vi "Z_HSw.vi"(8 "error in (no error)":errorcluster, 10 "Z_Source":T1, 11 "Z_HSw_in":refnum<class "Z_HSw.lvclass">) -> (0 "error out":errorcluster, 3 "Z_HSw_out":refnum<class "Z_HSw.lvclass">)   [LabVIEW 2019, in "Z_HSw.lvclass"]
uses:
  Z_HSw.lvclass
  ctl/Z_SourceInd.ctl
  ctl/Z_SourceIndL.ctl
  Z_source.ctl
  Z_HSw.lvclass/Z_HSw.ctl
  ctl/Z_HSw_state.ctl
  Timer Delay/Timers.lvlib
panel:
  out "Z1 ind":T2
  out "Z1 ind 2":T3
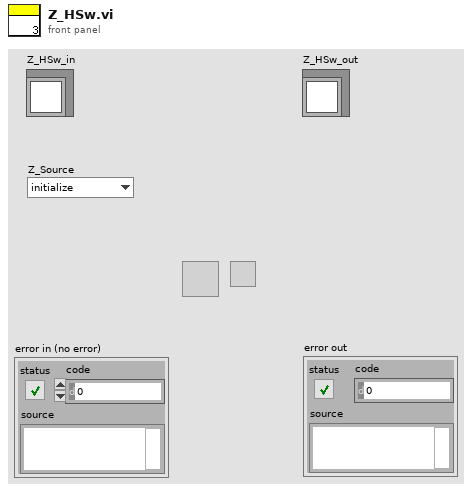
[diagram p1: front panel]
types:
  T1 = typedef "Z_source.ctl" = enum8{"initialize", "local disabled", "local hand", "hand", "auto", "dist"}
  T2 = typedef "Z_HSw.lvclass/Z_SourceIndL.ctl" = u8
  T3 = typedef "Z_HSw.lvclass/Z_SourceInd.ctl" = u8
  T4 = typedef "Z_HSw.lvclass/Z_HSw_state.ctl" = enum16{"init", "switch hand", "not hand", "hand", "switch auto", "not auto", "auto"}
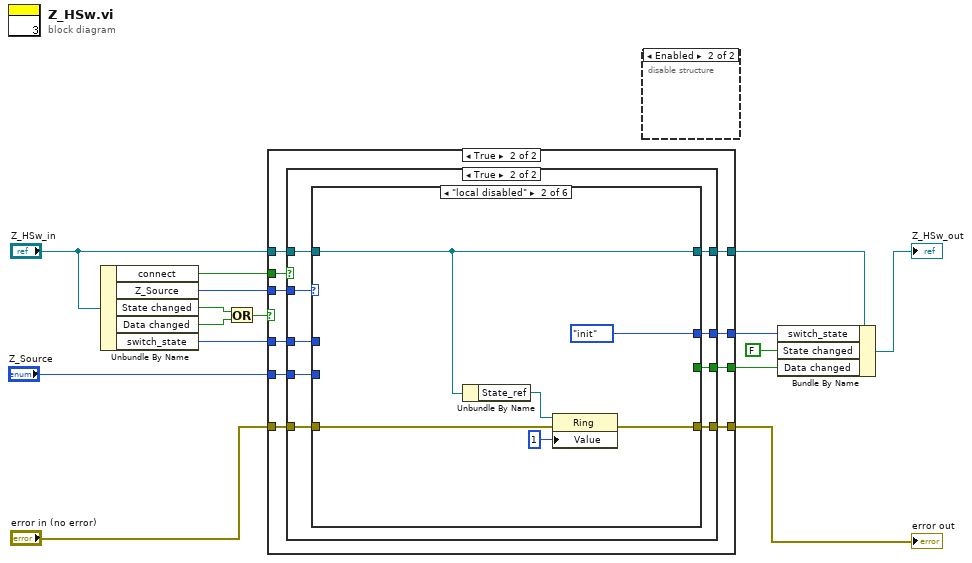
[diagram p0: block diagram]
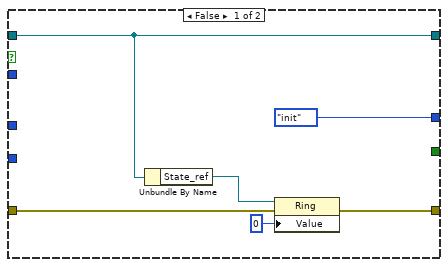
[diagram p3: hidden frame]
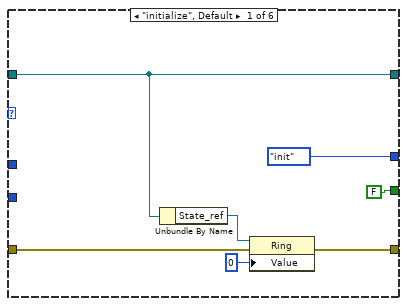
[diagram p4: hidden frame]
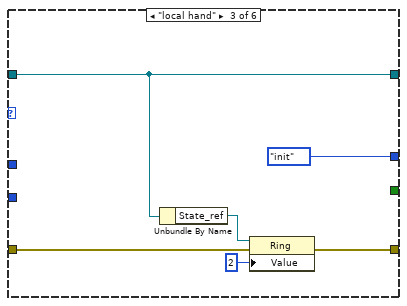
[diagram p5: hidden frame]
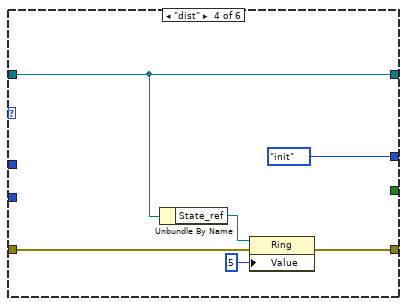
[diagram p6: hidden frame]
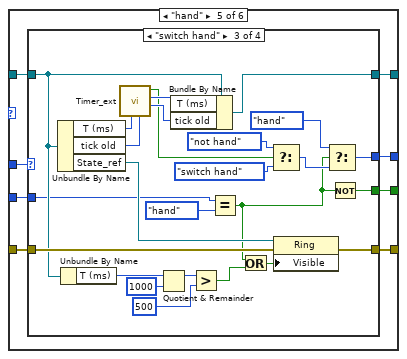
[diagram p7: hidden frame]
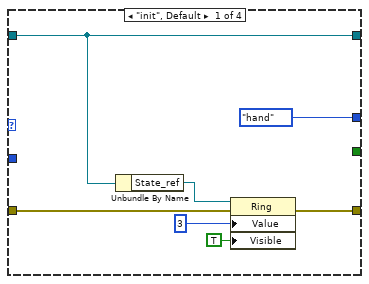
[diagram p8: hidden frame]
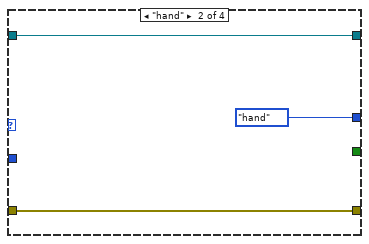
[diagram p9: hidden frame]
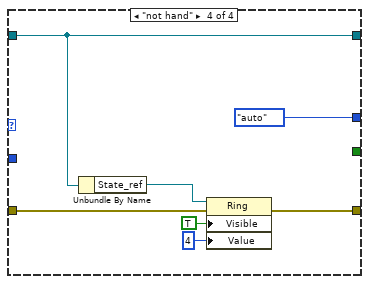
[diagram p10: hidden frame]
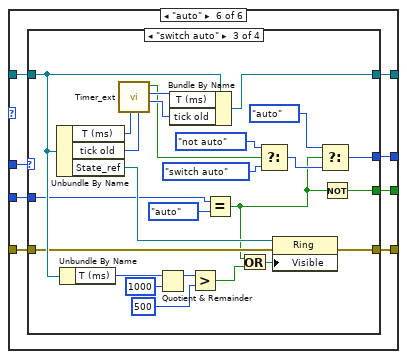
[diagram p11: hidden frame]
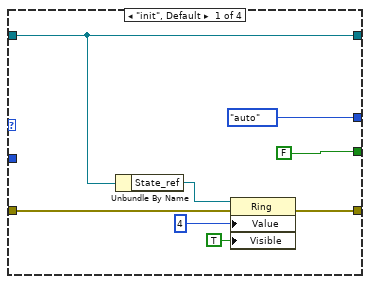
[diagram p12: hidden frame]
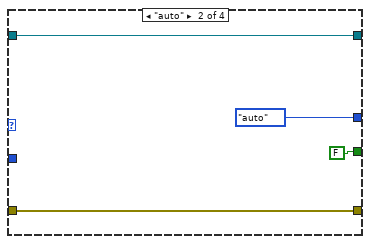
[diagram p13: hidden frame]
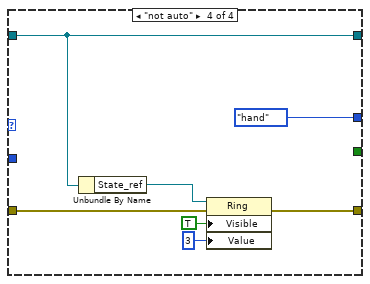
[diagram p14: hidden frame]
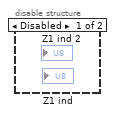
[diagram p15: hidden frame]
diagram:
  n1 = Unbundle By Name("Z_HSw_in") -> ("connect"=w10:bool, "Z_Source"=w9:T1, "State changed"=w5:bool, "Data changed"=w4:bool, "switch_state"=w3:T4)
  n2 = Or(x=w5, y=w4) -> (x .or. y?=w12:bool)
  n3 = case shown="True" w12 {
    tunnel: [w16 w28] -> w6
    tunnel: "error in (no error)" -> [w17 w27]
    tunnel: [w17 w26] -> w13
    tunnel: [w18 w25] -> w7
    tunnel: w10 -> [_ w24]
    tunnel: "Z_HSw_in" -> [w18 w23]
    tunnel: w9 -> [_ w22]
    tunnel: w3 -> [w16 w21]
    tunnel: [_ w20] -> w2
    tunnel: "Z_Source" -> [_ w19]
    frame False {
    }
    frame True {
      n4 = case shown="True" w24 {
        tunnel: w22 -> [_ w43]
        tunnel: [w29 w40] -> w25
        tunnel: [Z_HSw_state."init" ("switch_state") w42] -> w28
        tunnel: w27 -> [w30 w39]
        tunnel: w23 -> [w29 w41]
        tunnel: [w31 w38] -> w26
        tunnel: w21 -> [_ w37]
        tunnel: [_ w36] -> w20
        tunnel: w19 -> [_ w35]
        frame False {
          n5 = Unbundle By Name(w29) -> ("State_ref"=w33:refnum<vi>)
          n6 = property on="Property Node" class="Ring"(reference=w33, error in=w30, "Value"=u8 0 ("Z1_ind visu")) -> (error out=w31:errorcluster)  [unwired: 1 out]
        }
        frame True {
          n7 = case shown="\"local disabled\"" w43 {
            tunnel: [Z_HSw_state."init" ("switch_state") Z_HSw_state."init" ("switch_state") Z_HSw_state."init" ("switch_state") Z_HSw_state."init" ("switch_state") w74 w124] -> w42
            tunnel: w41 -> [w46 w52 w58 w64 w75 w125]
            tunnel: [w46 w52 w58 w64 w76 w126] -> w40
            tunnel: w39 -> [w47 w53 w59 w65 w73 w123]
            tunnel: [w48 w54 w60 w66 w72 w122] -> w38
            tunnel: w37 -> [_ _ _ _ w71 w121]
            tunnel: [FALSE _ _ _ w70 w120] -> w36
            tunnel: w35 -> [_ _ _ _ w69 w119]
            frame "initialize", Default {
              # "local hand"
              n8 = Unbundle By Name(w46) -> ("State_ref"=w50:refnum<vi>)
              n9 = property on="Property Node" class="Ring"(reference=w50, error in=w47, "Value"=u8 0 ("Z1_ind visu")) -> (error out=w48:errorcluster)  [unwired: 1 out]
            }
            frame "local disabled" {
              # "local hand"
              n10 = Unbundle By Name(w52) -> ("State_ref"=w56:refnum<vi>)
              n11 = property on="Property Node" class="Ring"(reference=w56, error in=w53, "Value"=u8 1 ("Z1_ind visu")) -> (error out=w54:errorcluster)  [unwired: 1 out]
            }
            frame "local hand" {
              # "local hand"
              n12 = Unbundle By Name(w58) -> ("State_ref"=w62:refnum<vi>)
              n13 = property on="Property Node" class="Ring"(reference=w62, error in=w59, "Value"=u8 2 ("Z1_ind visu")) -> (error out=w60:errorcluster)  [unwired: 1 out]
            }
            frame "dist" {
              # "local hand"
              n14 = Unbundle By Name(w64) -> ("State_ref"=w68:refnum<vi>)
              n15 = property on="Property Node" class="Ring"(reference=w68, error in=w65, "Value"=u8 5 ("Z1_ind visu")) -> (error out=w66:errorcluster)  [unwired: 1 out]
            }
            frame "hand" {
              # "local hand"
              n16 = case shown="\"switch hand\"" w71 {
                tunnel: [w78 w85 w97 w112] -> w76
                tunnel: w75 -> [w78 w85 w96 w112]
                tunnel: [Z_HSw_state."hand" ("switch_state") Z_HSw_state."hand" ("switch_state") w94 Z_HSw_state."auto" ("switch_state")] -> w74
                tunnel: w73 -> [w81 w84 w111 w118]
                tunnel: [w82 w84 w110 w117] -> w72
                tunnel: [_ _ w89 _] -> w70
                tunnel: w69 -> [_ _ w92 _]
                frame "init", Default {
                  n17 = Unbundle By Name(w78) -> ("State_ref"=w83:refnum<vi>)
                  n18 = property on="Property Node" class="Ring"(reference=w83, error in=w81, "Value"=u8 3 ("Z1_ind visu"), "Visible"=TRUE) -> (error out=w82:errorcluster)  [unwired: 1 out]
                }
                frame "hand" {
                }
                frame "switch hand" {
                  n19 = Unbundle By Name(w96) -> ("T (ms)"=w101:u32, "tick old"=w100:u32, "State_ref"=w109:refnum<vi>)
                  n20 = Unbundle By Name(w96) -> ("T (ms)"=w105:u32)
                  n21 = call "Timer_ext.vi"("tick old"=w100, "t ms old"=w101) -> ("tick"=w98:u32, "t ms"=w99:u32, "End"=w95:bool)  [unwired: 7 in]
                  n22 = Quotient & Remainder(x=w105, y=u32 1000) -> (x-y*floor(x/y)=w108:u32)  [unwired: 1 out]
                  n23 = Bundle By Name(cluster=w96, "T (ms)"=w99, "tick old"=w98) -> (w97:refnum<class "Z_HSw.lvclass">)
                  n24 = Greater?(x=w108, y=u32 500) -> (0:w104:bool)
                  n25 = Equal?(x=w92, y=Z_source."hand") -> (x = y?=w87:bool)
                  n26 = Or(x=w87, y=w104) -> (x .or. y?=w88:bool)
                  n27 = Select(t=Z_HSw_state."not hand" ("switch_state"), s=w95, f=Z_HSw_state."switch hand" ("switch_state")) -> (s? t:f=w93:T4)
                  n28 = property on="Property Node" class="Ring"(reference=w109, error in=w111, "Visible"=w88) -> (error out=w110:errorcluster)  [unwired: 1 out]
                  n29 = Select(t=Z_HSw_state."hand" ("switch_state"), s=w87, f=w93) -> (s? t:f=w94:T4)
                  n30 = Not(x=w87) -> (.not. x?=w89:bool)
                }
                frame "not hand" {
                  n31 = Unbundle By Name(w112) -> ("State_ref"=w115:refnum<vi>)
                  n32 = property on="Property Node" class="Ring"(reference=w115, error in=w118, "Visible"=TRUE, "Value"=u8 4 ("Z1_ind visu")) -> (error out=w117:errorcluster)  [unwired: 1 out]
                }
              }
            }
            frame "auto" {
              # "local hand"
              n33 = case shown="\"switch auto\"" w121 {
                tunnel: [w129 w137 w147 w164] -> w126
                tunnel: w125 -> [w129 w137 w150 w164]
                tunnel: [Z_HSw_state."auto" ("switch_state") Z_HSw_state."auto" ("switch_state") w146 Z_HSw_state."hand" ("switch_state")] -> w124
                tunnel: w123 -> [w132 w135 w149 w170]
                tunnel: [w133 w135 w148 w169] -> w122
                tunnel: [FALSE ("Visible") FALSE ("Visible") w141 _] -> w120
                tunnel: w119 -> [_ _ w142 _]
                frame "init", Default {
                  n34 = Unbundle By Name(w129) -> ("State_ref"=w134:refnum<vi>)
                  n35 = property on="Property Node" class="Ring"(reference=w134, error in=w132, "Value"=u8 4 ("Z1_ind visu"), "Visible"=TRUE) -> (error out=w133:errorcluster)  [unwired: 1 out]
                }
                frame "auto" {
                }
                frame "switch auto" {
                  n36 = Unbundle By Name(w150) -> ("T (ms)"=w155:u32, "tick old"=w154:u32, "State_ref"=w163:refnum<vi>)
                  n37 = Unbundle By Name(w150) -> ("T (ms)"=w159:u32)
                  n38 = call "Timer_ext.vi"("tick old"=w154, "t ms old"=w155) -> ("tick"=w152:u32, "t ms"=w153:u32, "End"=w151:bool)  [unwired: 7 in]
                  n39 = Quotient & Remainder(x=w159, y=u32 1000) -> (x-y*floor(x/y)=w162:u32)  [unwired: 1 out]
                  n40 = Bundle By Name(cluster=w150, "T (ms)"=w153, "tick old"=w152) -> (w147:refnum<class "Z_HSw.lvclass">)
                  n41 = Greater?(x=w162, y=u32 500) -> (0:w158:bool)
                  n42 = Equal?(x=w142, y=Z_source."auto") -> (x = y?=w139:bool)
                  n43 = Or(x=w139, y=w158) -> (x .or. y?=w140:bool)
                  n44 = Select(t=Z_HSw_state."not auto" ("switch_state"), s=w151, f=Z_HSw_state."switch auto" ("switch_state")) -> (s? t:f=w145:T4)
                  n45 = property on="Property Node" class="Ring"(reference=w163, error in=w149, "Visible"=w140) -> (error out=w148:errorcluster)  [unwired: 1 out]
                  n46 = Select(t=Z_HSw_state."auto" ("switch_state"), s=w139, f=w145) -> (s? t:f=w146:T4)
                  n47 = Not(x=w139) -> (.not. x?=w141:bool)
                }
                frame "not auto" {
                  n48 = Unbundle By Name(w164) -> ("State_ref"=w167:refnum<vi>)
                  n49 = property on="Property Node" class="Ring"(reference=w167, error in=w170, "Visible"=TRUE, "Value"=u8 3 ("Z1_ind visu")) -> (error out=w169:errorcluster)  [unwired: 1 out]
                }
              }
            }
          }
        }
      }
    }
  }
  "error out" <- w13
  n50 = disable-structure shown="Enabled" {
    frame Disabled {
    }
    frame Enabled {
    }
  }
  n51 = Bundle By Name(cluster=w7, "switch_state"=w6, "State changed"=FALSE ("Data changed"), "Data changed"=w2) -> (→"Z_HSw_out":refnum<class "Z_HSw.lvclass">)
